vi "UniDaq32_OutBit.vi"(8 "error in (no error)":errorcluster, 10 "BL":bool, 11 "IO_Output":T1=enum."推出氣缸_3") -> (0 "error out":errorcluster)   [LabVIEW 2015]
uses:
  Ctrl/UniDaq_SelectOutPut.ctl
  Ctrl/IO Card_Type.ctl
  global/IO_ClassTypeData.vi
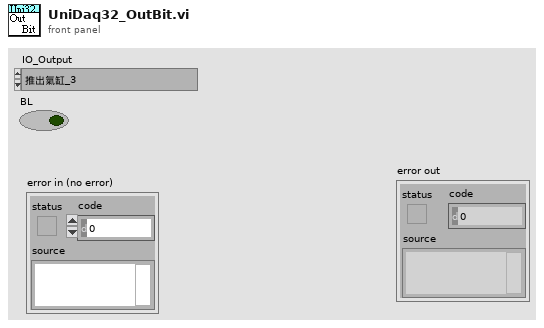
[diagram p1: front panel]
types:
  T1 = typedef "UniDaq_SelectOutPut.ctl" = enum16{"進料閘門氣缸", "進料翻轉氣缸", "UBE#1", "UBE#2", "探針夾持氣缸", "Bar Code Scanner啟動", "儀器啟動", "UBE#3", "UBE#4", "電池旋轉移載氣缸", "UBE#5", "UBE#6", "不良品排出分料氣缸", "不良品排出上下分層氣缸", "UBE#7", "UBE#8", "不良品排出氣缸", "UBE#9", "UBE#10", "推出氣缸_1", "推出氣缸_2", "推出氣缸_3", "推出氣缸_4", "推出氣缸_5", "推出氣缸_6", "推出氣缸_7", "UBE#11", "UBE#12", "移入軌道氣缸#模組一", "軌道分料氣缸#模組一", "移入旋轉台氣缸#模組一", "旋轉台氣缸#模組一", "UBE#13", "UBE#14", "移入軌道氣缸#模組二", "軌道分料氣缸#模組二", "移入旋轉台氣缸#模組二", "旋轉台氣缸#模組二", "UBE#15", "UBE#16", "移入軌道氣缸#模組三", "軌道分料氣缸#模組三", "移入旋轉台氣缸#模組三", "旋轉台氣缸#模組三", "UBE#17", "UBE#18", "移入軌道氣缸#模組四", "軌道分料氣缸#模組四", "移入旋轉台氣缸#模組四", "旋轉台氣缸#模組四", "UBE#19", "UBE#20", "移入軌道氣缸#模組五", "軌道分料氣缸#模組五", "移入旋轉台氣缸#模組五", "旋轉台氣缸#模組五", "UBE#21", "UBE#22", "移入軌道氣缸#模組六", "軌道分料氣缸#模組六", "移入旋轉台氣缸#模組六", "旋轉台氣缸#模組六", "UBE#23", "UBE#24"}
  T2 = typedef "IO Card_Type.ctl" = enum16{"None", "Unidaq32", "IPC_3005(9700)", "6480", "2410C-64", "Zan"}
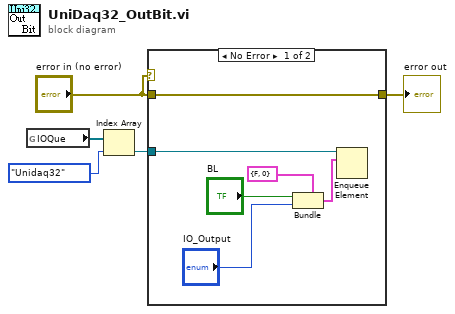
[diagram p0: block diagram]
diagram:
  n1 = global read "IO_ClassTypeData.vi" "IOQue"() -> (w3:refnum<queue>[])
  n2 = Index Array(array=w3, index=IO_Card_Type."Unidaq32" ("IO Card Type")) -> (element=w1:refnum<queue>)
  n3 = case shown="No Error" "error in (no error)" {
    tunnel: "error in (no error)" -> [w6 w12]
    tunnel: [w6 w12] -> w5
    tunnel: w1 -> [w11 _]
    frame No Error {
      n4 = Bundle(cluster=cluster{"BL":bool, "Index":i32} {"BL"=FALSE, "Index"=0} ("element"), "BL"="BL", "Index"="IO_Output") -> (w8:cluster{"BL":bool, "Index":i32})
      n5 = Enqueue Element(queue=w11, element=w8) -> ()  [unwired: 2 in, 3 out]
    }
    frame Error {
    }
  }
  "error out" <- w5
